vi "render_overlay_elements.vi"(6 "Image Overlay (extras from control loop)":T2[](array[typedef]) {"Drawing Mode" items=["Frame", "Fill", "Highlight"]}, 7 "Image":T1) -> (3 "Image Out":T1)   [LabVIEW 2010]
uses:
  <vilib>/vision/Image Controls.llb/IMAQ Image.ctl
  overlay_element.ctl
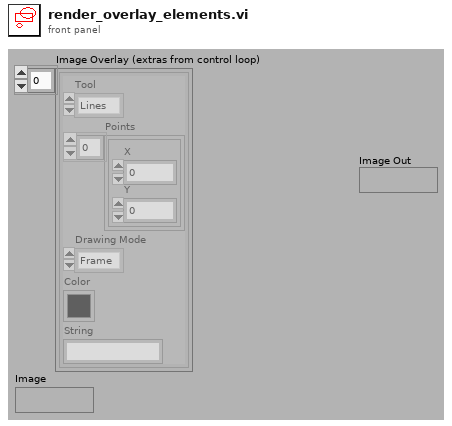
[diagram p1: front panel]
types:
  T1 = typedef "IMAQ Image.ctl" = refnum<image>
  T2 = typedef "overlay_element.ctl" = cluster{"Tool":enum16{"Lines", "Oval", "Rectangle", "Text"}, "Points":cluster{"X":dbl, "Y":dbl}[], "Drawing Mode":u32, "Color":u32, "String":string}
  T3 = cluster{"Desired Font (Application)":enum16{"User-specified Font", "Application Font", "System Font", "Dialog Font"}, "[User-specified Font]":cluster{"Font Name":string, "Size":i16, "Strikeout?":bool, "Italic?":bool, "Underline?":bool, "Outline?":bool, "Shadow?":bool, "Bold?":bool, "Rotation Angle":dbl}, "Horizontal Alignment":i16, "Vertical Alignment":i16}
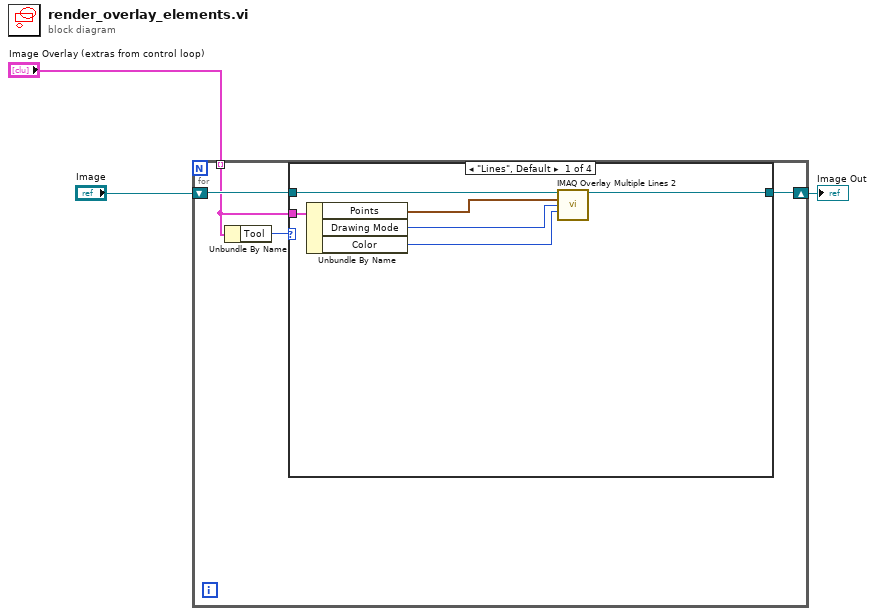
[diagram p0: block diagram]
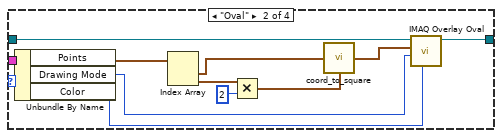
[diagram p2: hidden frame]
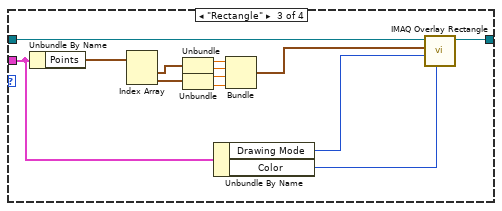
[diagram p3: hidden frame]
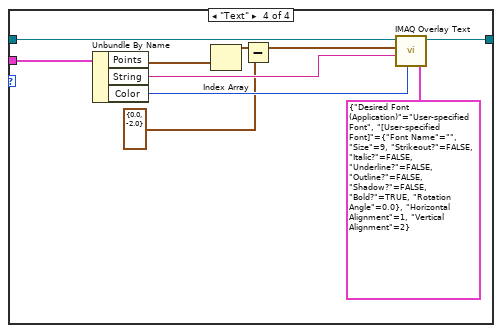
[diagram p4: hidden frame]
diagram:
  n1 = for {
    tunnel: "Image Overlay (extras from control loop)" -> [w4] mode=indexing
    shift-right: [w5] -> w1
    shift-left: "Image" -> [w6]
    n2 = Unbundle By Name(w4) -> ("Tool"=w7:enum16{"Lines", "Oval", "Rectangle", "Text"})
    n3 = case shown="\"Lines\", Default" w7 {
      tunnel: w6 -> [w13 w23 w36 w46]
      tunnel: [w12 w24 w37 w47] -> w5
      tunnel: w4 -> [w11 w21 w28 w45]
      frame "Lines", Default {
        n4 = Unbundle By Name(w11) -> ("Points"=w8:cluster{"X":dbl, "Y":dbl}[], "Drawing Mode"=w10:u32, "Color"=w9:u32)
        n5 = call "IMAQ Overlay Multiple Lines 2"("Image"=w13, "Line End Points"=w8, "Drawing Mode (Frame)"=w10, "Color"=w9) -> ("Image Out"=w12:T1)  [unwired: 10 in, 1 out]
      }
      frame "Oval" {
        n6 = Unbundle By Name(w21) -> ("Points"=w20:cluster{"X":dbl, "Y":dbl}[], "Drawing Mode"=w16:u32, "Color"=w15:u32)
        n7 = Index Array(array=w20) -> (element #1=w14:cluster{"X":dbl, "Y":dbl}, element #2=w19:cluster{"X":dbl, "Y":dbl})  [unwired: 2 in]
        n8 = Multiply(x=w19, y=2) -> (x*y=w18:cluster{"X":dbl, "Y":dbl})
        n9 = call "coord_to_square.vi"("Size"=w18, "Centre"=w14) -> ("rectangle"=w22:cluster{dbl, dbl, dbl, dbl})  [unwired: 2 in]
        n10 = call "IMAQ Overlay Oval"("Color"=w15, "Drawing Mode (Frame)"=w16, "Bounding Rectangle"=w22, "Image"=w23) -> ("Image Out"=w24:T1)  [unwired: 6 in, 1 out]
      }
      frame "Rectangle" {
        n11 = Unbundle By Name(w28) -> ("Points"=w25:cluster{"X":dbl, "Y":dbl}[])
        n12 = Index Array(array=w25) -> (element #1=w35:cluster{"X":dbl, "Y":dbl}, element #2=w34:cluster{"X":dbl, "Y":dbl})  [unwired: 2 in]
        n13 = Unbundle(w35) -> ("X"=w33:dbl, "Y"=w32:dbl)
        n14 = Unbundle(w34) -> ("X"=w31:dbl, "Y"=w30:dbl)
        n15 = Unbundle By Name(w28) -> ("Drawing Mode"=w27:u32, "Color"=w26:u32)
        n16 = Bundle("X"=w33, "Y"=w32, "X"=w31, "Y"=w30) -> (w29:cluster{"X":dbl, "Y":dbl, "X":dbl, "Y":dbl})  [unwired: 1 in]
        n17 = call "IMAQ Overlay Rectangle"("Color"=w26, "Drawing Mode (Frame)"=w27, "Rectangle"=w29, "Image"=w36) -> ("Image Out"=w37:T1)  [unwired: 6 in, 1 out]
      }
      frame "Text" {
        n18 = Unbundle By Name(w45) -> ("Points"=w44:cluster{"X":dbl, "Y":dbl}[], "String"=w43:string, "Color"=w42:u32)
        n19 = Index Array(array=w44) -> (element=w41:cluster{"X":dbl, "Y":dbl})  [unwired: 1 in]
        n20 = Subtract(x=w41, y=cluster{"X":dbl, "Y":dbl} {"X"=0.0, "Y"=-2.0}) -> (x-y=w39:cluster{"X":dbl, "Y":dbl})
        n21 = call "IMAQ Overlay Text"("Text Color (black)"=w42, "Font, Size & Style"=T3 {"Desired Font (Application)"=enum."User-specified Font", "[User-specified Font]"={"Font Name"="", "Size"=9, "Strikeout?"=FALSE, "Italic?"=FALSE, "Underline?"=FALSE, "Outline?"=FALSE, "Shadow?"=FALSE, "Bold?"=TRUE, "Rotation Angle"=0.0}, "Horizontal Alignment"=1, "Vertical Alignment"=2}, "String"=w43, "Origin"=w39, "Image"=w46) -> ("Image Out"=w47:T1)  [unwired: 5 in, 1 out]
      }
    }
  }
  "Image Out" <- w1
